vi "Handle Command.vi"(8 "error in (no error)":errorcluster, 9 "Value":bool, 11 "Valve in":refnum<class "ValveControl.lvclass">) -> (0 "error out":errorcluster, 3 "Valve out":refnum<class "ValveControl.lvclass">)   [LabVIEW 2020, in "VolatusControl.lvlib" / "ValveControl.lvclass"]
uses:
  ValveControl.lvclass
  ValveControl.lvclass/ValveControl.ctl
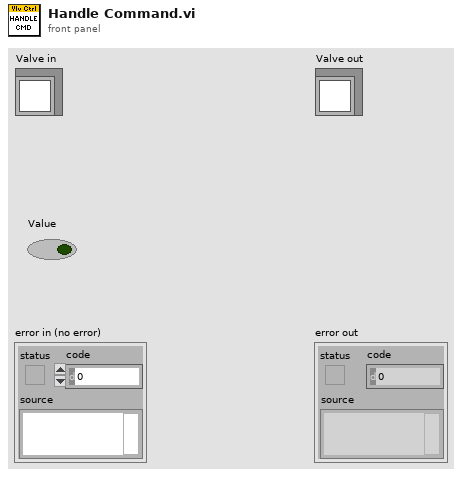
[diagram p1: front panel]
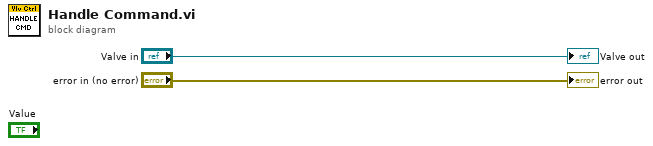
[diagram p0: block diagram]
diagram:
  "error out" <- "error in (no error)"
  "Valve out" <- "Valve in"
